vi "AddBus.vi"(8 "ErrorArray In":errorcluster[](array[cluster]), 10 "EvtReg":refnum<event-registration>, 11 "NISTBusClass In":refnum<class "NISTBus.lvclass">) -> (0 "ErrorArray Out":errorcluster[](array[cluster]), 2 "EvtReg":refnum<event-registration>, 3 "NISTBusClass Out":refnum<class "NISTBus.lvclass">)   [LabVIEW 2014, in "Bus.lvlib" / "NISTBus.lvclass"]
uses:
  NISTBus.lvclass
  <userlib>/NIST/NISTErrorLib/NISTErrorLib.lvlib
  FGenModule/FGenModule.lvlib
  WfrmGenerator/WfrmModule/WfrmModule.lvlib
  Framework/TestFramework.lvlib
  Bus.lvlib
  <userlib>/NIST/ModuleAdminLib/ModuleAdmin/ModuleAdmin.lvclass
  WfrmGenerator/WfrmModule/Protected/Broadcasts/clBroadcastEvents.ctl
  WfrmGenerator/WfrmModule/Protected/clEventType.ctl
  FGenModule/Protected/Broadcasts/clBroadcastEvents.ctl
  FGenModule/Protected/clEventType.ctl
  Framework/UserEvents/Protected/clUserEventType.ctl
  Framework/UserEvents/Protected/Requests/clRequestEvents.ctl
panel:
  # "If you want to add other Broadcast Events, open this typedef, copy an existing event and rename it to your event name.\n\nNext create an \"arg\" typedef for the  data and put it into PublicAPI/Arguments/Broadcasts\n\nAfter that, you will need to create a new roadcast vi in Protected/Broadcast.  Look at DidInit.vi or the reportError.vi as examples."
  # "If you want to add other Broadcast Events, open this typedef, copy an existing event and rename it to your event name.\n\nNext create a typedef for the  data and put it into PublicAPI/Arguments/Broadcasts"
  # "If you want to add other Broadcast Events, open this typedef, copy an existing event and rename it to your event name.\n\nNext create an \"arg\" typedef for the  data and put it into PublicAPI/Arguments/Broadcasts\n\nAfter that, you will need to create a new roadcast vi in Protected/Broadcast.  Look at DidInit.vi or the reportError.vi as examples."
  # "If you want to add other Broadcast Events, open this typedef, copy an existing event and rename it to your event name.\n\nNext create a typedef for the  data and put it into PublicAPI/Arguments/Broadcasts"
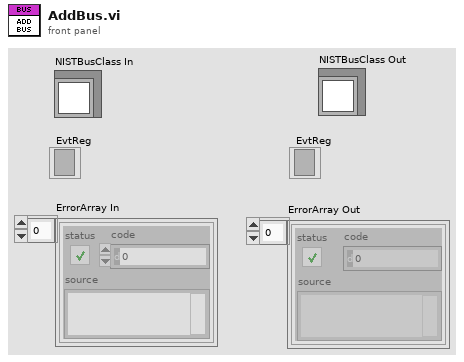
[diagram p1: front panel]
types:
  T1 = typedef "WfrmModule.lvlib/clBroadcastEvents.ctl" = cluster{"DidInit":refnum<user-event>, "StatusUpdate":refnum<user-event>, "ErrorReport":refnum<user-event>, "DidStop":refnum<user-event>, "ReadEvtConfig":refnum<user-event>, "ReadTimeArray":refnum<user-event>, "ReadEvtParams":refnum<user-event>, "GetEvtReportArray":refnum<user-event>, "ReadPathToPlugin":refnum<user-event>, "GetEvtSignal":refnum<user-event>, "SendArbWfrm":refnum<user-event>}
  T2 = typedef "FGenModule.lvlib/clBroadcastEvents.ctl" = cluster{"DidInit":refnum<user-event>, "StatusUpdate":refnum<user-event>, "ErrorReport":refnum<user-event>, "DidStop":refnum<user-event>, "PathToINI":refnum<user-event>, "ChannelName":refnum<user-event>, "ArbWfrmConfig":refnum<user-event>}
  T3 = typedef "TestFramework.lvlib/clFrameworkData.ctl" = cluster{"NISTBusClassInstances":refnum<class "NISTBus.lvclass">[], "NISTFGenINIFilePaths":path[], "NISTWfrmINIFilePaths":path[]}
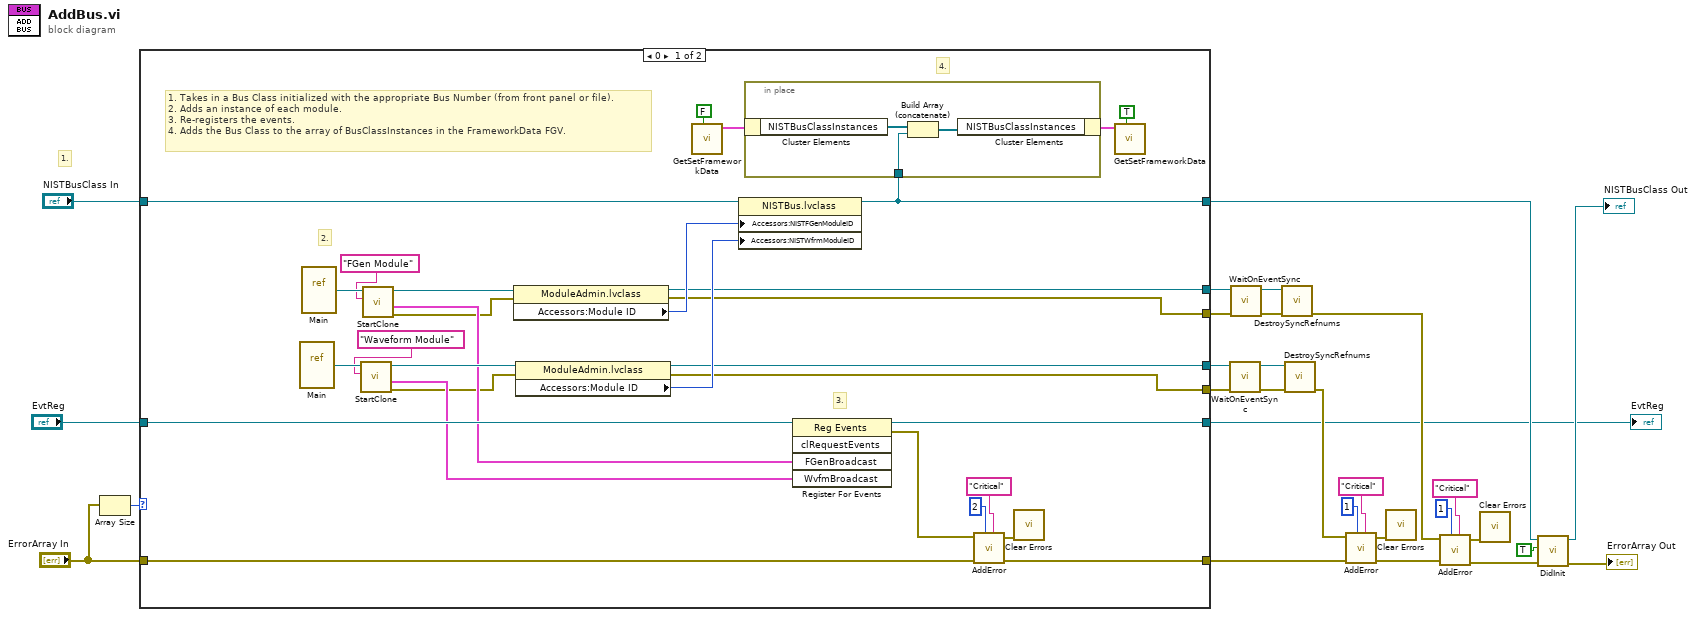
[diagram p0: block diagram]
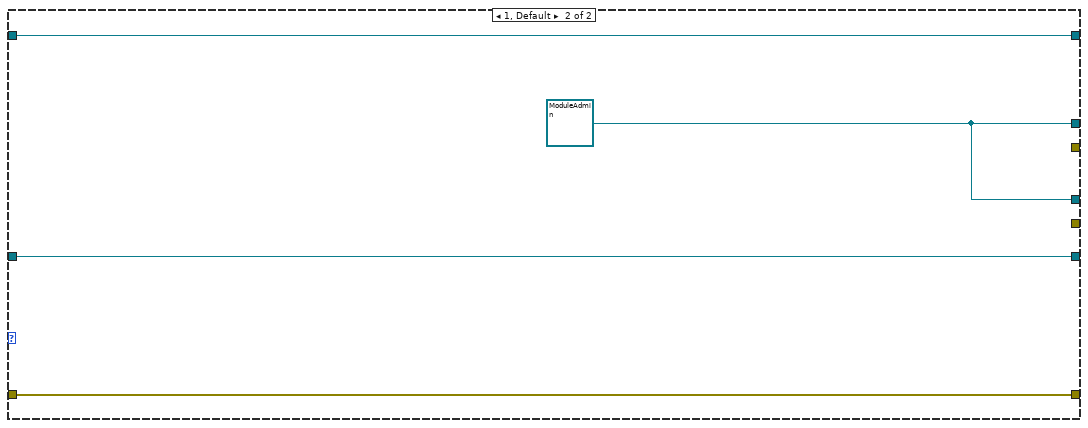
[diagram p2: hidden frame]
diagram:
  # "1."
  n1 = Array Size(array="ErrorArray In") -> (size(s)=w28:i32)
  n2 = case shown="0" w28 {
    tunnel: "ErrorArray In" -> [w55 w64]
    tunnel: "EvtReg" -> [w48 w63]
    tunnel: "NISTBusClass In" -> [w43 w62]
    tunnel: [w39 w65] -> w23
    tunnel: [w38 w65] -> w20
    tunnel: [w37 _] -> w19
    tunnel: [w36 _] -> w18
    tunnel: [w35 w64] -> w10
    tunnel: [w34 w63] -> w1
    tunnel: [w29 w62] -> w4
    frame 0 {
      # "4."
      # "3."
      # "2."
      # "1. Takes in a Bus Class initialized with the appropriate Bus Number (from front panel or file).\n2. Adds an instance of each module.\n3. Re-registers the events.\n4. Adds the Bus Class to the array of BusClassInstances in the FrameworkData FGV."
      n3 = vi-ref "Main.vi"() -> (w53:refnum<vi>)
      n4 = vi-ref "Main.vi"() -> (w54:refnum<vi>)
      n5 = call "StartClone.vi"("ModuleName"="Waveform Module", "VI Refnum"=w53) -> ("error out"=w44:errorcluster, "WvfrmEvents"=w46:T1, "ModuleAdmin"=w49:refnum<class "ModuleAdmin.lvclass">)  [unwired: 7 in]
      n6 = call "StartClone.vi"("ModuleName"="FGen Module", "VI Refnum"=w54) -> ("error out"=w45:errorcluster, "FGenBroadcast"=w47:T2, "ModuleAdmin"=w50:refnum<class "ModuleAdmin.lvclass">)  [unwired: 7 in]
      n7 = property class="ModuleAdmin.lvclass"(reference=w50, error in=w45) -> (reference out=w38:refnum<class "ModuleAdmin.lvclass">, error out=w36:errorcluster, "Accessors:Module ID"=w42:i32)
      n8 = property class="ModuleAdmin.lvclass"(reference=w49, error in=w44) -> (reference out=w39:refnum<class "ModuleAdmin.lvclass">, error out=w37:errorcluster, "Accessors:Module ID"=w41:i32)
      n9 = call "GetSetFrameworkData.vi"("Set (F)"=FALSE) -> ("clFrameworkData Out"=w32:T3)  [unwired: 10 in]
      n10 = property class="NISTBus.lvclass"(reference=w43, "Accessors:NISTFGenModuleID"=w42, "Accessors:NISTWfrmModuleID"=w41) -> (reference out=w29:refnum<class "NISTBus.lvclass">)  [unwired: 1 in, 1 out]
      n11 = in-place {
        in-place-border: w29 -> [w60]
        n12 = in-place-cluster #1(w32) -> ("NISTBusClassInstances"=w61:refnum<class "NISTBus.lvclass">[])
        n13 = Build Array (concatenate)(w61, w60) -> (w59:refnum<class "NISTBus.lvclass">[])
        n14 = in-place-cluster #1("NISTBusClassInstances"=w59) -> (w31:T3)
      }
      n15 = register-events(reference=w48, w47, w46) -> (reference out=w34:refnum<event-registration>, error out=w40:errorcluster)  [unwired: 2 in]
      n16 = call <userlib>:"AddError.vi"("Severity"="Critical" ("String"), "Priority"=u8 2, "ErrorArray"=w55, "error in (no error)"=w40) -> ("ErrorArray"=w35:errorcluster[], "error out"=w58:errorcluster)  [unwired: 6 in]
      n17 = call <vilib>:"Clear Errors.vi"("error in (no error)"=w58) -> ()  [unwired: 5 in, 2 out]
      n18 = call "GetSetFrameworkData.vi"("Set (F)"=TRUE, "clFrameworkData In"=w31) -> ()  [unwired: 9 in, 1 out]
    }
    frame 1, Default {
      w65 = refnum<class "ModuleAdmin.lvclass"> refnum ("ModuleAdmin.lvlib:ModuleAdmin.lvclass")
    }
  }
  "EvtReg" <- w1
  n19 = call <userlib>:"WaitOnEventSync.vi"("error in (no error)"=w19, "ModuleAdmin"=w23) -> ("error out"=w25:errorcluster, "ModuleAdmin"=w24:refnum<class "ModuleAdmin.lvclass">)  [unwired: 8 in]
  n20 = call <userlib>:"WaitOnEventSync.vi"("error in (no error)"=w18, "ModuleAdmin"=w20) -> ("error out"=w21:errorcluster, "ModuleAdmin"=w22:refnum<class "ModuleAdmin.lvclass">)  [unwired: 8 in]
  n21 = call <userlib>:"DestroySyncRefnums.vi"("error in (no error)"=w21, "ModuleAdmin"=w22) -> ("error out"=w8:errorcluster)  [unwired: 9 in]
  n22 = call <userlib>:"DestroySyncRefnums.vi"("error in (no error)"=w25, "ModuleAdmin"=w24) -> ("error out"=w11:errorcluster)  [unwired: 9 in]
  n23 = call <userlib>:"AddError.vi"("Severity"="Critical" ("String"), "Priority"=u8 1, "ErrorArray"=w10, "error in (no error)"=w11) -> ("ErrorArray"=w9:errorcluster[], "error out"=w17:errorcluster)  [unwired: 6 in]
  n24 = call <vilib>:"Clear Errors.vi"("error in (no error)"=w17) -> ()  [unwired: 5 in, 2 out]
  n25 = call <userlib>:"AddError.vi"("Severity"="Critical" ("String"), "Priority"=u8 1, "ErrorArray"=w9, "error in (no error)"=w8) -> ("ErrorArray"=w6:errorcluster[], "error out"=w14:errorcluster)  [unwired: 6 in]
  n26 = call <vilib>:"Clear Errors.vi"("error in (no error)"=w14) -> ()  [unwired: 5 in, 2 out]
  n27 = call "DidInit.vi"("ErrorArray In"=w6, "Init?"=TRUE, "NISTBus In"=w4) -> ("ErrorArray Out"=→"ErrorArray Out":errorcluster[], "NISTBus Out"=→"NISTBusClass Out":refnum<class "NISTBus.lvclass">)  [unwired: 7 in]
